vi "ygdll path.vi"(8 "error in (no error)":errorcluster) -> (0 "error out":errorcluster, 3 "appended path":path)   [LabVIEW 2023]
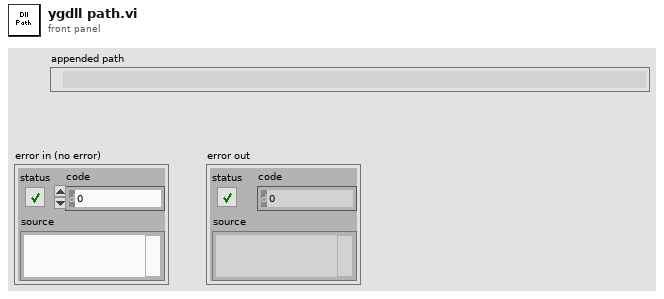
[diagram p1: front panel]
types:
  T1 = enum32{"invalid app kind", "Development System", "Run Time System", "Student Edition", "Embedded LabVIEW", "Evaluation", "Custom"}
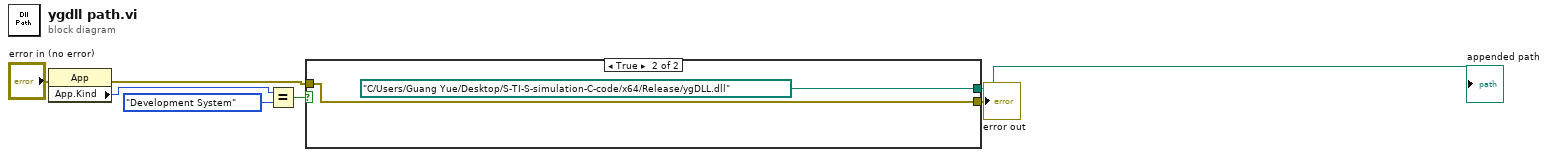
[diagram p0: block diagram]
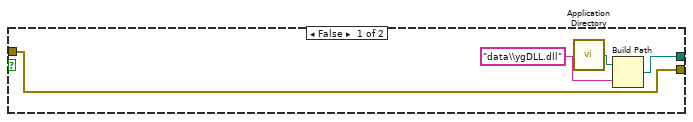
[diagram p2: hidden frame]
diagram:
  n1 = property class="App"(error in="error in (no error)") -> (error out=w5:errorcluster, "App.Kind"=w2:T1)  [unwired: 1 in, 1 out]
  n2 = Equal?(x=w2, y=T1."Development System" ("Application:Kind")) -> (x = y?=w4:bool)
  n3 = case shown="True" w4 {
    tunnel: [w9 path "C:/Users/Guang Yue/Desktop/S-TI-S-simulation-C-code/x64/Release/ygDLL.dll"] -> w6
    tunnel: w5 -> [w8 w12]
    tunnel: [w8 w12] -> w7
    frame False {
      n4 = call <vilib>:"Application Directory.vi"() -> ("Application Directory"=w11:path)
      n5 = Build Path(base path=w11, name or relative path="data\\ygDLL.dll") -> (appended path=w9:path)
    }
    frame True {
    }
  }
  "error out" <- w7
  "appended path" <- w6
